vi "micUnbundle_III.vi"(0 "422nm Data":T2, 5 "532nm Data":T3, 7 "785nm Data":T4) -> (4 "Output Cluster":T1, 6 "422 New Array":dbl[](array[numeric]), 8 "532 New Array":dbl[](array[numeric]), 10 "785 New Array":dbl[](array[numeric]))   [LabVIEW 2011]
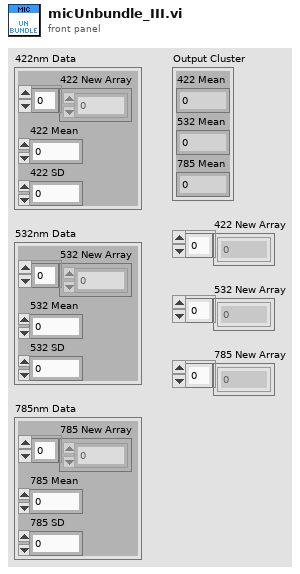
[diagram p1: front panel]
types:
  T1 = cluster{"422 Mean":dbl, "532 Mean":dbl, "785 Mean":dbl}
  T2 = cluster{"422 New Array":dbl[], "422 Mean":dbl, "422 SD":dbl}
  T3 = cluster{"532 New Array":dbl[], "532 Mean":dbl, "532 SD":dbl}
  T4 = cluster{"785 New Array":dbl[], "785 Mean":dbl, "785 SD":dbl}
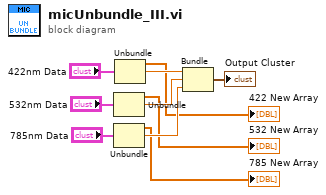
[diagram p0: block diagram]
diagram:
  n1 = Unbundle("532nm Data") -> ("532 New Array"=→"532 New Array":dbl[], "532 Mean"=w5:dbl)  [unwired: 1 out]
  n2 = Unbundle("785nm Data") -> ("785 New Array"=→"785 New Array":dbl[], "785 Mean"=w6:dbl)  [unwired: 1 out]
  n3 = Unbundle("422nm Data") -> ("422 New Array"=→"422 New Array":dbl[], "422 Mean"=w4:dbl)  [unwired: 1 out]
  n4 = Bundle("422 Mean"=w4, "532 Mean"=w5, "785 Mean"=w6) -> (→"Output Cluster":T1)  [unwired: 1 in]
